vi "build.from.objects.vi"(11 "volume objects":cluster{"Array":T2[]}[](array[cluster])) -> (0 "total issues":i32, 1 "collection count":i32, 2 "Report":T1[](array[typedef]) {"cover_date" format="%<%x>T"}, 3 "Exported Report":string[][](array[string]))   [LabVIEW 2024]
uses:
  CV_Shared_Library/volume.object--cluster.ctl
  CV_Shared_Library/volume.type--enum.ctl
  comic_manager/TypeDefs/issue.display--cluster.ctl
  report.issue--cluster.ctl
  CV_Shared_Library/CV_Shared_Library.lvlib
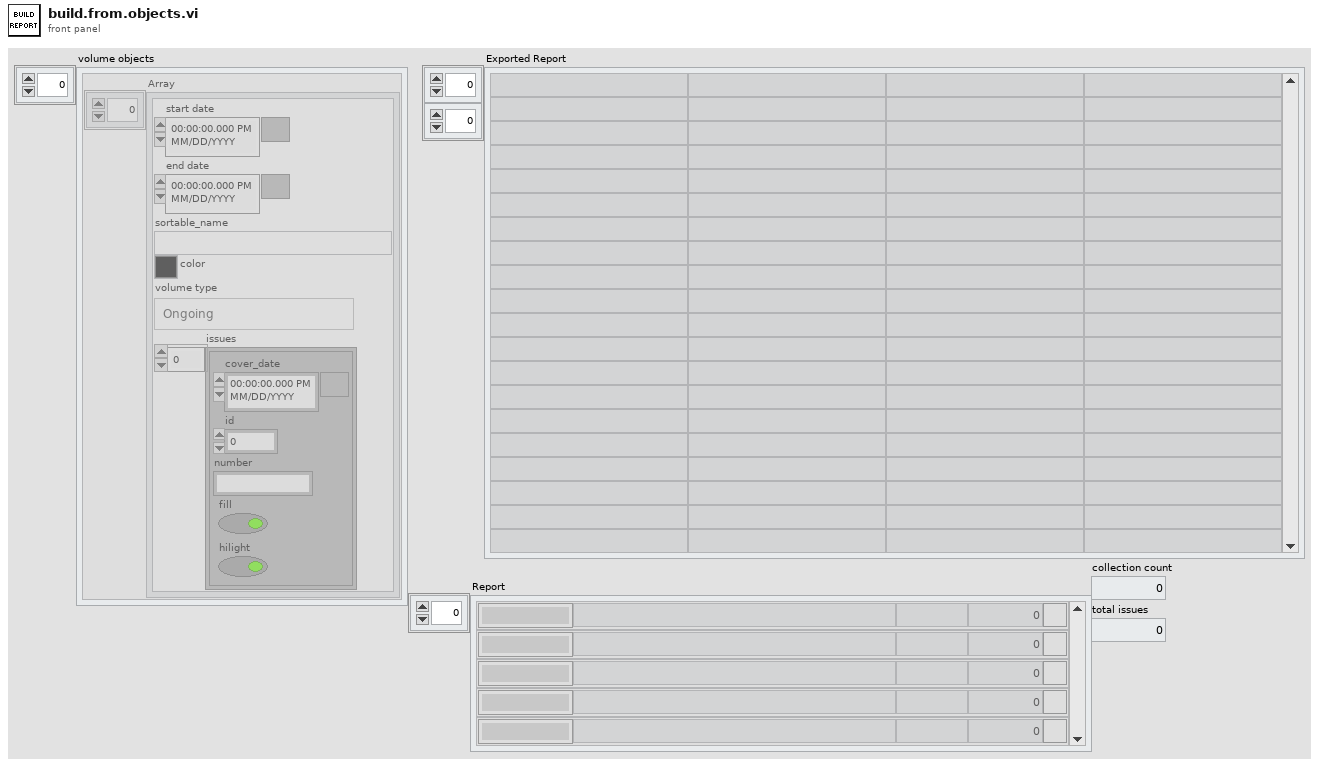
[diagram p1: front panel]
types:
  T1 = typedef "report.issue--cluster.ctl" = cluster{"cover_date":timestamp, "sortable_name":string, "number":string, "id":i32, "hilight":bool}
  T2 = typedef "CV_Shared_Library.lvlib/volume.object--cluster.ctl" = cluster{"start date":timestamp, "end date":timestamp, "sortable_name":string, "color":u32, "volume type":T3, "issues":T4[]}
  T3 = typedef "CV_Shared_Library.lvlib/volume.type--enum.ctl" = enum16{"Ongoing", "Limited Series", "Annual", "One Shot", "Reprint/Document", "Star Comics", "Epic Comics"}
  T4 = typedef "CV_Shared_Library.lvlib/issue.display--cluster.ctl" = cluster{"cover_date":timestamp, "id":i32, "number":string, "fill":bool, "hilight":bool}
  T5 = cluster{"cover_date":timestamp, "result string":string, "number":string, "id":i32, "hilight":bool}
  T6 = cluster{"cover_date":timestamp, "result string":string, "number":string, "id":i32, "hilight":bool}[]
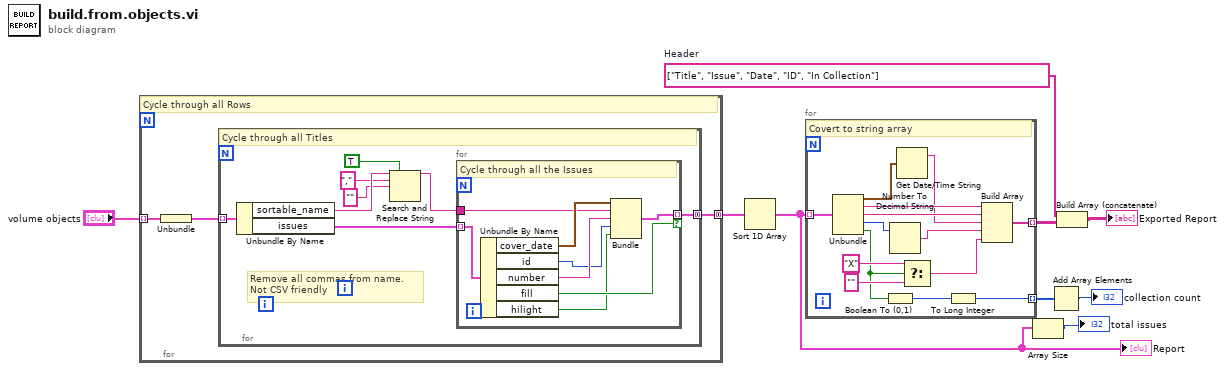
[diagram p0: block diagram]
diagram:
  w6 = string[] ["Title", "Issue", "Date", "ID", "In Collection"]  # Header
  n1 = for {
    tunnel: "volume objects" -> [w12] mode=indexing
    tunnel: [w10] -> w8 mode=concatenating
    # "Cycle through all Rows"
    n2 = Unbundle(w12) -> ("Array"=w11:T2[])
    n3 = for {
      tunnel: w11 -> [w20] mode=indexing
      tunnel: [w18] -> w10 mode=concatenating
      # "Remove all commas from name.\nNot CSV friendly"
      # "Cycle through all Titles"
      n4 = Unbundle By Name(w20) -> ("sortable_name"=w17:string, "issues"=w19:T4[])
      n5 = Search and Replace String(replace all?=TRUE ("replace all? (F)"), input string=w17, search string=",", replace string="" ("replace string (\"\")")) -> (result string=w13:string)  [unwired: 4 in, 3 out]
      n6 = for {
        tunnel: w19 -> [w28] mode=indexing
        tunnel: w13 -> [w26]
        tunnel: [w23] -> w18 mode=indexing if=w22
        # "Cycle through all the Issues"
        n7 = Unbundle By Name(w28) -> ("cover_date"=w27:timestamp, "id"=w24:i32, "number"=w25:string, "fill"=w22:bool, "hilight"=w21:bool)
        n8 = Bundle("cover_date"=w27, "result string"=w26, "number"=w25, "id"=w24, "hilight"=w21) -> (w23:T5)  [unwired: 1 in]
      }
    }
  }
  n9 = Sort 1D Array(array=w8) -> (sorted array=w3:T6)
  "Report" <- w3
  n10 = for {
    tunnel: w3 -> [w42] mode=indexing
    tunnel: [w35] -> w7 mode=indexing
    tunnel: [w29] -> w4 mode=indexing
    # "Covert to string array"
    n11 = Unbundle(w42) -> ("cover_date"=w41:timestamp, "result string"=w40:string, "number"=w39:string, "id"=w38:i32, "hilight"=w31:bool)
    n12 = Boolean To (0,1)(Boolean=w31) -> (0, 1=w30:i16)
    n13 = Number To Decimal String(number=w38) -> (decimal integer string=w37:string)  [unwired: 1 in]
    n14 = Get Date/Time String(seconds (now)=w41) -> (date string=w36:string)  [unwired: 2 in, 1 out]
    n15 = Select(t="X", s=w31, f="") -> (s? t:f=w32:string)
    n16 = To Long Integer(number=w30) -> (32bit integer=w29:i32)
    n17 = Build Array(w40, w39, w36, w37, w32) -> (w35:string[])
  }
  n18 = Array Size(array=w3) -> (size(s)=→"total issues":i32)
  n19 = Add Array Elements(numeric array=w4) -> (sum=→"collection count":i32)
  n20 = Build Array (concatenate)(w6, w7) -> (→"Exported Report":string[][])
